vi "Init.vi"(8 "error in (no error)":errorcluster) -> (0 "error out":errorcluster, 3 "VMR out":refnum<class "VMR.lvclass">)   [LabVIEW 2022 SP3, in "VMR-Deck.lvlib" / "VMR.lvclass"]
uses:
  VMR.lvclass
  VMR.lvclass/VMR.ctl
  <vilib>/IlluminatedG/IG VoicemeeterRemote API/VoiceMeeterRemote/VoiceMeeterRemote/VoiceMeeterRemote.lvclass
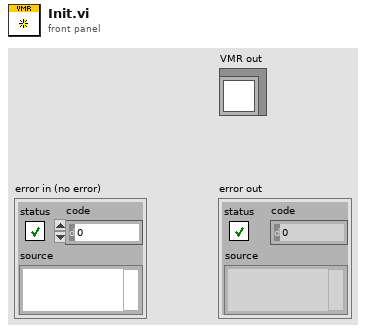
[diagram p1: front panel]
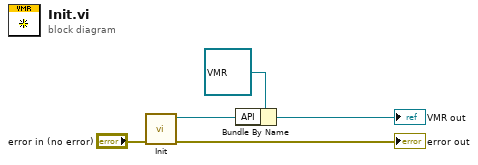
[diagram p0: block diagram]
diagram:
  n1 = call <vilib>:"Init.vi"("error in (no error)"="error in (no error)") -> ("error out"=→"error out":errorcluster, "VoiceMeeterRemote out"=w2:refnum<class "VoiceMeeterRemote.lvclass">)  [unwired: 8 in, 1 out]
  n2 = Bundle By Name(cluster=refnum<class "VMR.lvclass"> refnum ("VMR in"), "API"=w2) -> (→"VMR out":refnum<class "VMR.lvclass">)
